vi "Fill Function (SubVI).vi"(0 "Signals IN":T2={"Dispense"=FALSE, "Fill"=FALSE, "Spray"=FALSE, "Drain"=TRUE, "Complete"=FALSE, "Fill Error"=FALSE, "Disp. Error"=FALSE, "Fill Timeout"=FALSE, "Disp. Timeout"=FALSE, "Purge"=TRUE}, 1 "Values IN":T3 {"Drain Time (s)" format="%.2f"; "Drain Rate (g/sec)" format="%.2f"}, 2 "FILL Setpoint (g)":dbl, 3 "Measured Mass (g)":dbl(knob) scale=0.0..1000.0, 4 "Settings":T1={"ON Settings"={"Enable Dynamic Setpoint?"=TRUE, "Enable Dynamic Dispense Time?"=TRUE, "Enable Drain Rate Functions"=TRUE, "Dispense Sample Time (s)"=0.1, "Mass Average Samples"=20, "ON Timeout (sec)"=300.0, "1st Setpoint (% of Target)"=90.0, "2nd Setpoint (% of Target)"=95.0, "3rd Setpoint (% of Target)"=100.0, "Measure Dispense Delay (sec)"=10.0, "Minimum Spray Time (s)"=2.0, "Pump Reverse Time (s)"=10.0}, "OFF Settings"={"Drain Sample Time (s)"=0.1, "Drain Rate Ave Size"=100, "Drain Rate Limits (± g/sec)"=100.0, "Level Slope Range (± g/sec)"=0.05, "OFF Timeout (sec)"=300.0, "Near SP Slope Level (± g/sec)"=0.005, "Near Setpoint Threshold (%)"=99.0}, "Overshoot Settings"={"Time Limit (s)"=30.0, "Container MAX (g)"=1500.0, "Max FILL Slope (+/- g/sec)"=100.0, "% Overshot to Enable (>)"=3.0}, "FILL Timeout (s)"=300.0, "Full \nSettle Time (s)"=30.0, "Pre-Hydrate \nSpray Time (s)"=0.0, "Pre-Hydrate \nWait Time (s)"=10.0, "m Value "=1.0, "b Value"=0.0, "Enable Overshoot Adjust?"=FALSE} {"ON Settings"."Pump Reverse Time (s)" min=0.0 max=60.0; "OFF Settings"."Near SP Slope Level (± g/sec)" format="%.3g"; "OFF Settings"."Level Slope Range (± g/sec)" format="%.3g"}, 9 "Main Case Change?":bool) -> (14 "Signals OUT":T2={"Dispense"=FALSE, "Fill"=FALSE, "Spray"=FALSE, "Drain"=TRUE, "Complete"=FALSE, "Fill Error"=FALSE, "Disp. Error"=FALSE, "Fill Timeout"=FALSE, "Disp. Timeout"=FALSE, "Purge"=TRUE}, 15 "Values OUT":T3 {"Drain Time (s)" format="%.2f"; "Drain Rate (g/sec)" format="%.2f"}, 19 "Fill FN Complete":bool)   [LabVIEW 2011]
panel:
  # "ONLY ADJUST\nBOLD VALUES!"
  # "Corrected Mass = SDC Mass * m + b"
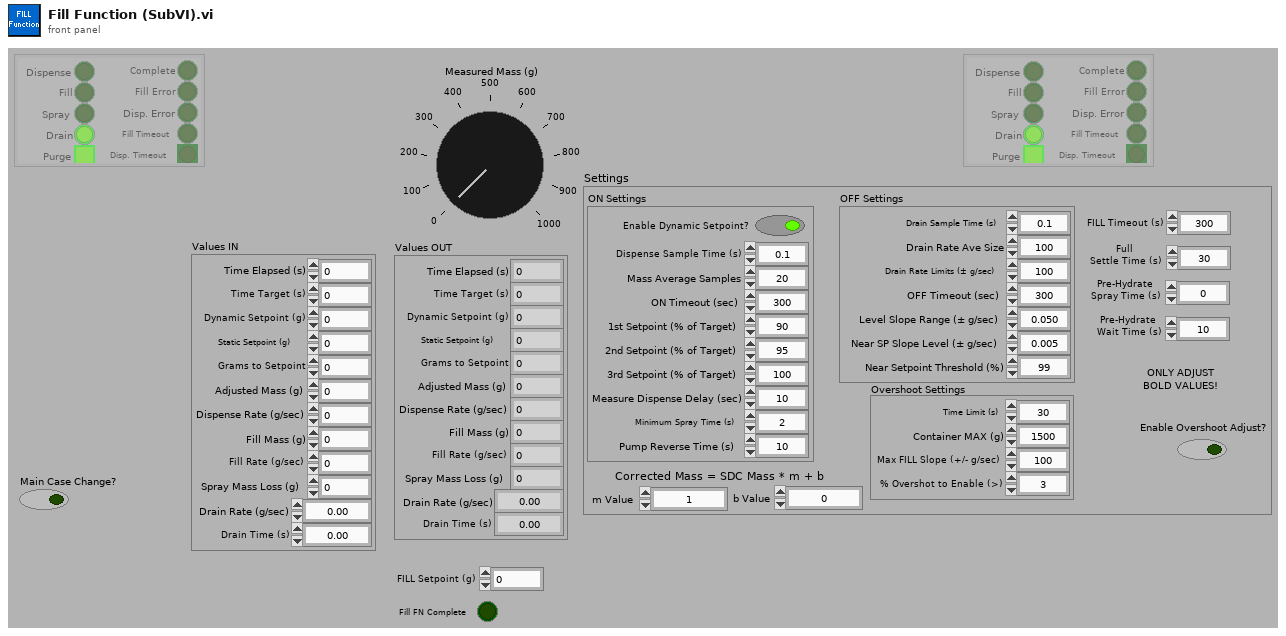
[diagram p1: front panel]
types:
  T1 = cluster{"ON Settings":cluster{"Enable Dynamic Setpoint?":bool, "Enable Dynamic Dispense Time?":bool, "Enable Drain Rate Functions":bool, "Dispense Sample Time (s)":dbl, "Mass Average Samples":i32, "ON Timeout (sec)":dbl, "1st Setpoint (% of Target)":dbl, "2nd Setpoint (% of Target)":dbl, "3rd Setpoint (% of Target)":dbl, "Measure Dispense Delay (sec)":dbl, "Minimum Spray Time (s)":dbl, "Pump Reverse Time (s)":dbl}, "OFF Settings":cluster{"Drain Sample Time (s)":dbl, "Drain Rate Ave Size":i32, "Drain Rate Limits (± g/sec)":dbl, "Level Slope Range (± g/sec)":dbl, "OFF Timeout (sec)":dbl, "Near SP Slope Level (± g/sec)":dbl, "Near Setpoint Threshold (%)":dbl}, "Overshoot Settings":cluster{"Time Limit (s)":dbl, "Container MAX (g)":dbl, "Max FILL Slope (+/- g/sec)":dbl, "% Overshot to Enable (>)":dbl}, "FILL Timeout (s)":dbl, "Full \nSettle Time (s)":dbl, "Pre-Hydrate \nSpray Time (s)":dbl, "Pre-Hydrate \nWait Time (s)":dbl, "m Value ":dbl, "b Value":dbl, "Enable Overshoot Adjust?":bool}
  T2 = cluster{"Dispense":bool, "Fill":bool, "Spray":bool, "Drain":bool, "Complete":bool, "Fill Error":bool, "Disp. Error":bool, "Fill Timeout":bool, "Disp. Timeout":bool, "Purge":bool}
  T3 = cluster{"Time Elapsed (s)":dbl, "Time Target (s)":dbl, "Dynamic Setpoint (g)":dbl, "Static Setpoint (g)":dbl, "Grams to Setpoint":dbl, "Adjusted Mass (g)":dbl, "Dispense Rate (g/sec)":dbl, "Fill Mass (g)":dbl, "Fill Rate (g/sec)":dbl, "Spray Mass Loss (g)":dbl, "Drain Rate (g/sec)":dbl, "Drain Time (s)":dbl}
  T4 = enum16{"FILL INITIAL", "FILL ACTIVE", "POST FILL WAIT", "HYDRATION SPRAY", "POST HYDRATE WAIT", "FILL COMPLETE"}
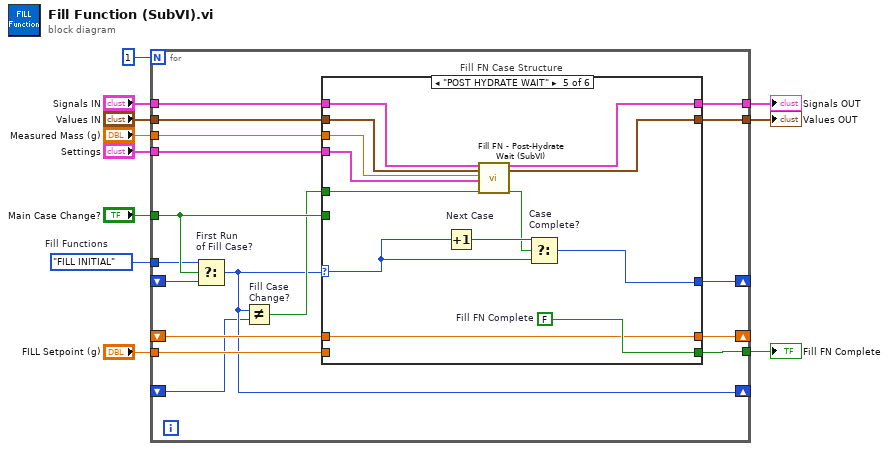
[diagram p0: block diagram]
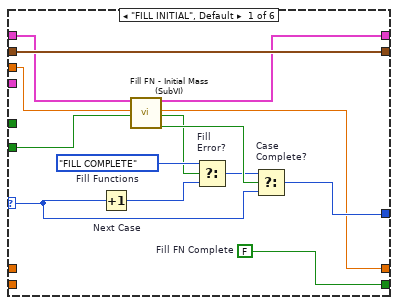
[diagram p2: hidden frame]
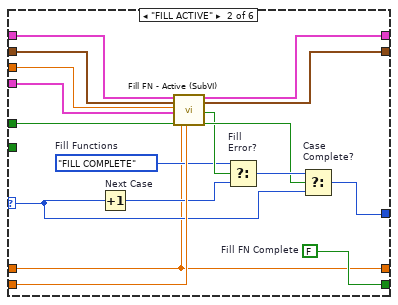
[diagram p3: hidden frame]
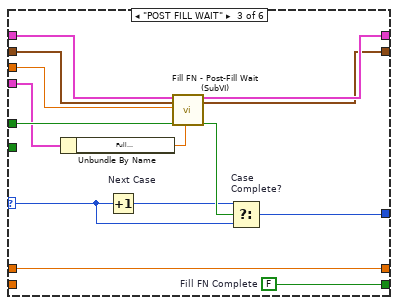
[diagram p4: hidden frame]
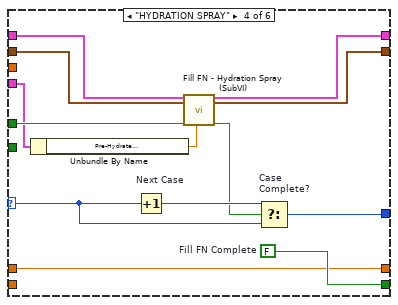
[diagram p5: hidden frame]
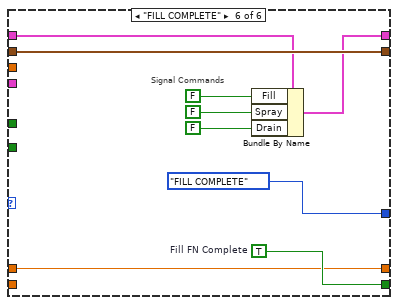
[diagram p6: hidden frame]
diagram:
  w4 = T4."FILL INITIAL"  # Fill Functions
  n1 = for {
    N: 1 -> [_]
    shift-right: [w27] -> _
    shift-left: _ -> [w28]
    tunnel: "Main Case Change?" -> [w26]
    shift-right: [w14] -> _
    shift-left: _ -> [w13]
    shift-right: [w16] -> _
    shift-left: _ -> [w20]
    tunnel: "Measured Mass (g)" -> [w24]
    tunnel: "Signals IN" -> [w23]
    tunnel: [w22] -> w2
    tunnel: "Settings" -> [w21]
    tunnel: "FILL Setpoint (g)" -> [w19]
    tunnel: "Values IN" -> [w18]
    tunnel: [w17] -> w8
    tunnel: [w15] -> w7
    tunnel: w4 -> [w12]
    n2 = Select "First Run\nof Fill Case?"(t=w12, s=w26, f=w28) -> (s? t:f=w14:T4)
    n3 = Not Equal? "Fill Case\nChange?"(x=w14, y=w13) -> (x != y?=w25:bool)
    n4 = case "Fill FN Case Structure" shown="\"POST HYDRATE WAIT\"" w14 {
      selector: w14 -> [w38 w46 w68 w79 w93 _]
      tunnel: [w37 w57 w69 w80 w91 T4."FILL COMPLETE" ("Fill Functions")] -> w27
      tunnel: w26 -> [w30 _ _ _ _ _]
      tunnel: w25 -> [_ w56 w70 w82 w95 _]
      tunnel: w24 -> [w29 w52 w71 _ w89 _]
      tunnel: w23 -> [w32 w54 w73 w86 w99 w101]
      tunnel: [w31 w50 w72 w85 w98 w100] -> w22
      tunnel: w21 -> [_ w43 w61 w75 w88 _]
      tunnel: [w35 w49 w66 w83 w97 w108] -> w17
      tunnel: w20 -> [_ w44 w62 w76 w87 w105]
      tunnel: w19 -> [_ w53 _ _ _ _]
      tunnel: w18 -> [w35 w51 w67 w84 w96 w108]
      tunnel: [w33 w44 w62 w76 w87 w105] -> w16
      tunnel: [w34 w55 w63 w77 w90 w107] -> w15
      frame "FILL INITIAL", Default {
        w34 = FALSE  # Fill FN Complete
        w42 = T4."FILL COMPLETE"  # Fill Functions
        n5 = Increment "Next Case"(x=w38) -> (x+1=w41:T4)
        n6 = call "Fill FN - Initial Mass (SubVI).vi"("Signals IN"=w32, "Measured Mass (g)"=w29, "Main Case Change?"=w30) -> ("Signals OUT"=w31:T2, "Initial Mass"=w33:dbl, "Fill Error"=w36:bool, "Case Complete"=w40:bool)  [unwired: 1 in, 12 out]
        n7 = Select "Fill \nError?"(t=w42, s=w36, f=w41) -> (s? t:f=w39:T4)
        n8 = Select "Case\nComplete?"(t=w39, s=w40, f=w38) -> (s? t:f=w37:T4)
      }
      frame "FILL ACTIVE" {
        w47 = T4."FILL COMPLETE"  # Fill Functions
        w55 = FALSE  # Fill FN Complete
        n9 = Increment "Next Case"(x=w46) -> (x+1=w45:T4)
        n10 = call "Fill FN - Active (SubVI).vi"("Signals IN"=w54, "Values IN"=w51, "Measured Mass (g)"=w52, "Settings"=w43, "Fill Case Change?"=w56, "Initial Mass (g)"=w44, "FILL Setpoint (g)"=w53) -> ("Signals OUT"=w50:T2, "Values OUT"=w49:T3, "Fill Timeout"=w48:bool, "Case Complete"=w58:bool)  [unwired: 1 in, 8 out]
        n11 = Select "Fill \nError?"(t=w47, s=w48, f=w45) -> (s? t:f=w59:T4)
        n12 = Select "Case\nComplete?"(t=w59, s=w58, f=w46) -> (s? t:f=w57:T4)
      }
      frame "POST FILL WAIT" {
        w63 = FALSE  # Fill FN Complete
        n13 = Unbundle By Name(w61) -> ("Full \nSettle Time (s)"=w60:dbl)
        n14 = Increment "Next Case"(x=w68) -> (x+1=w64:T4)
        n15 = call "Fill FN - Post-Fill Wait (SubVI).vi"("Signals IN"=w73, "Values IN"=w67, "Measured Mass (g)"=w71, "Fill Case Change?"=w70, "Full \nSettle Time (s)"=w60) -> ("Signals OUT"=w72:T2, "Values OUT"=w66:T3, "Case Complete"=w65:bool)  [unwired: 1 in, 11 out]
        n16 = Select "Case\nComplete?"(t=w64, s=w65, f=w68) -> (s? t:f=w69:T4)
      }
      frame "HYDRATION SPRAY" {
        w77 = FALSE  # Fill FN Complete
        n17 = Unbundle By Name(w75) -> ("Pre-Hydrate \nSpray Time (s)"=w74:dbl)
        n18 = Increment "Next Case"(x=w79) -> (x+1=w81:T4)
        n19 = call "Fill FN - Hydration Spray (SubVI).vi"("Signals IN"=w86, "Values IN"=w84, "Fill Case Change?"=w82, "Pre-Hydrate \nSpray Time (s)"=w74) -> ("Signals OUT"=w85:T2, "Values OUT"=w83:T3, "Case Complete"=w78:bool)  [unwired: 1 in, 12 out]
        n20 = Select "Case\nComplete?"(t=w81, s=w78, f=w79) -> (s? t:f=w80:T4)
      }
      frame "POST HYDRATE WAIT" {
        w90 = FALSE  # Fill FN Complete
        n21 = Increment "Next Case"(x=w93) -> (x+1=w94:T4)
        n22 = call "Fill FN - Post-Hydrate Wait (SubVI).vi"("Signals IN"=w99, "Values IN"=w96, "Measured Mass (g)"=w89, "Settings"=w88, "Fill Case Change?"=w95) -> ("Signals OUT"=w98:T2, "Values OUT"=w97:T3, "Case Complete"=w92:bool)  [unwired: 12 out]
        n23 = Select "Case\nComplete?"(t=w94, s=w92, f=w93) -> (s? t:f=w91:T4)
      }
      frame "FILL COMPLETE" {
        w107 = TRUE  # Fill FN Complete
        # "Signal Commands"
        n24 = Bundle By Name(cluster=w101, "Fill"=FALSE, "Spray"=FALSE, "Drain"=FALSE) -> (w100:T2)
      }
    }
  }
  "Fill FN Complete" <- w7
  "Values OUT" <- w8
  "Signals OUT" <- w2
